vi "T.vi"(2 "S":bool, 3 "T":bool, 4 "R":bool) -> (0 "!Q":bool, 1 "Q":bool)   [LabVIEW 2013]
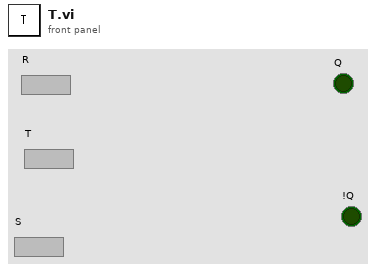
[diagram p1: front panel]
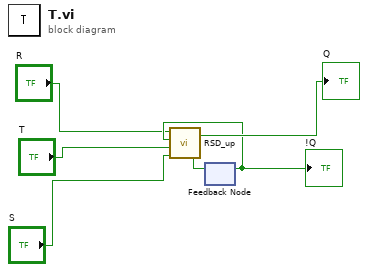
[diagram p0: block diagram]
diagram:
  n1 = feedback #1() -> (w4:bool)  [unwired: 1 in]
  "!Q" <- w4
  n2 = call "RSD_up.vi"("S"="S", "C"="T", "D"=w4, "R"="R") -> ("!Q"=w5:bool, "Q"=→"Q":bool)
  n3 = feedback-in #1(w5) -> ()
